vi "Periodic Tasks.vi"(8 "error in":errorcluster) -> ()   [LabVIEW 2019]
doc: "This VI runs in parallel to other tasks. It can contain as many user-defined periodic loops as you need. These can carry out PID or other sorts of timed response."
uses:
  <vilib>/Rock Robotics/WPI/DriverStation/WPI_DriverStationRobotMode2.ctl
  <vilib>/Rock Robotics/WPI/Utilities/WPI_GetSetVariantRefNum.vi
  <vilib>/Rock Robotics/Network Tables/NT Read Boolean.vi
  Robot Global Data.vi
  <vilib>/Rock Robotics/Network Tables/NT Write Boolean.vi
  <vilib>/Rock Robotics/Network Tables/NT Write Number.vi
  <vilib>/Rock Robotics/WPI/RobotDrive/WPI_RobotDriveArcadeDrive_Standard(NoSaturation).vi
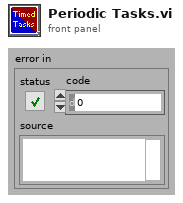
[diagram p1: front panel]
types:
  T1 = typedef "WPI_JoystickDevRef.ctl" = cluster{"Device":T2}
  T2 = typedef "WPI_JoystickDeviceEnum.ctl" = enum16{"USB 0", "USB 1", "USB 2", "USB 3", "USB 4", "USB 5"}
  T3 = typedef "WPI_RobotDriveDevRef.ctl" = cluster{"DevStatus":errorcluster, "Motors[]":T4[], "Square Inputs":bool, "Max Output":dbl}
  T4 = typedef "WPI_MotorControlDeviceRef.ctl" = cluster{"DeviceStatus":errorcluster, "Type":T5, "PWM":cluster{"PWM Channel":T6, "DeadBand":T7}, "CAN":cluster{"Device Number":u8, "SetOutput VI Ref":variant, "GetOutput VI Ref":variant, "Enable VI Ref":variant, "Disable VI Ref":variant, "Data":variant}, "Invert":bool, "DIO PWM":cluster{"PWM \"Enable\" Channel":T6, "DIOChannel":T8, "PWM Rate":dbl}}
  T5 = typedef "WPI_MotorControlType.ctl" = enum16{"PWM", "CAN", "DIO PWM"}
  T6 = typedef "FPGA_DIOPWMChannel.ctl" = enum8{"PWM 0", "PWM 1", "PWM 2", "PWM 3", "PWM 4", "PWM 5", "PWM 6", "PWM 7", "PWM 8", "PWM 9", "PWM MXP 0", "PWM MXP 1", "PWM MXP 2", "PWM MXP 3", "PWM MXP 4", "PWM MXP 5", "PWM MXP 6", "PWM MXP 7", "PWM MXP 8", "PWM MXP 9", "Invalid"}
  T7 = typedef "WPI_PWMDeadband.ctl" = cluster{"Name":string, "maxPositivePwm":i32, "minPositivePwm":i32, "centerPwm":i32, "maxNegativePwm":i32, "minNegativePwm":i32, "angularRange":u16}
  T8 = typedef "FPGA_DIOChannel.ctl" = enum8{"DIO 0", "DIO 1", "DIO 2", "DIO 3", "DIO 4", "DIO 5", "DIO 6", "DIO 7", "DIO 8", "DIO 9", "DIO MXP 0", "DIO MXP 1", "DIO MXP 2", "DIO MXP 3", "DIO MXP 4", "DIO MXP 5", "DIO MXP 6", "DIO MXP 7", "DIO MXP 8", "DIO MXP 9", "DIO MXP 10", "DIO MXP 11", "DIO MXP 12", "DIO MXP 13", "DIO MXP 14", "DIO MXP 15", "SPI Port CS1", "SPI Port CS2", "SPI Port CS3", "SPI Port MISO", "SPI Port MOSI", "Invalid"}
  T9 = cluster{"JoystickDevRef":T1, "RobotDriveDevRef":T3}
  T10 = typedef "WPI_DriverStationRobotMode2.ctl" = enum16{"Autonomous Disabled", "Autonomous Enabled", "Teleop Disabled", "Teleop Enabled", "Disconnected", "Finish", "Test Disabled", "Test Enabled", "Emergency Stopped"}
  T11 = typedef "WPI_ServoDeviceRef.ctl" = cluster{"DeviceStatus":errorcluster, "PWM Channel":T6, "DeadBand":T7}
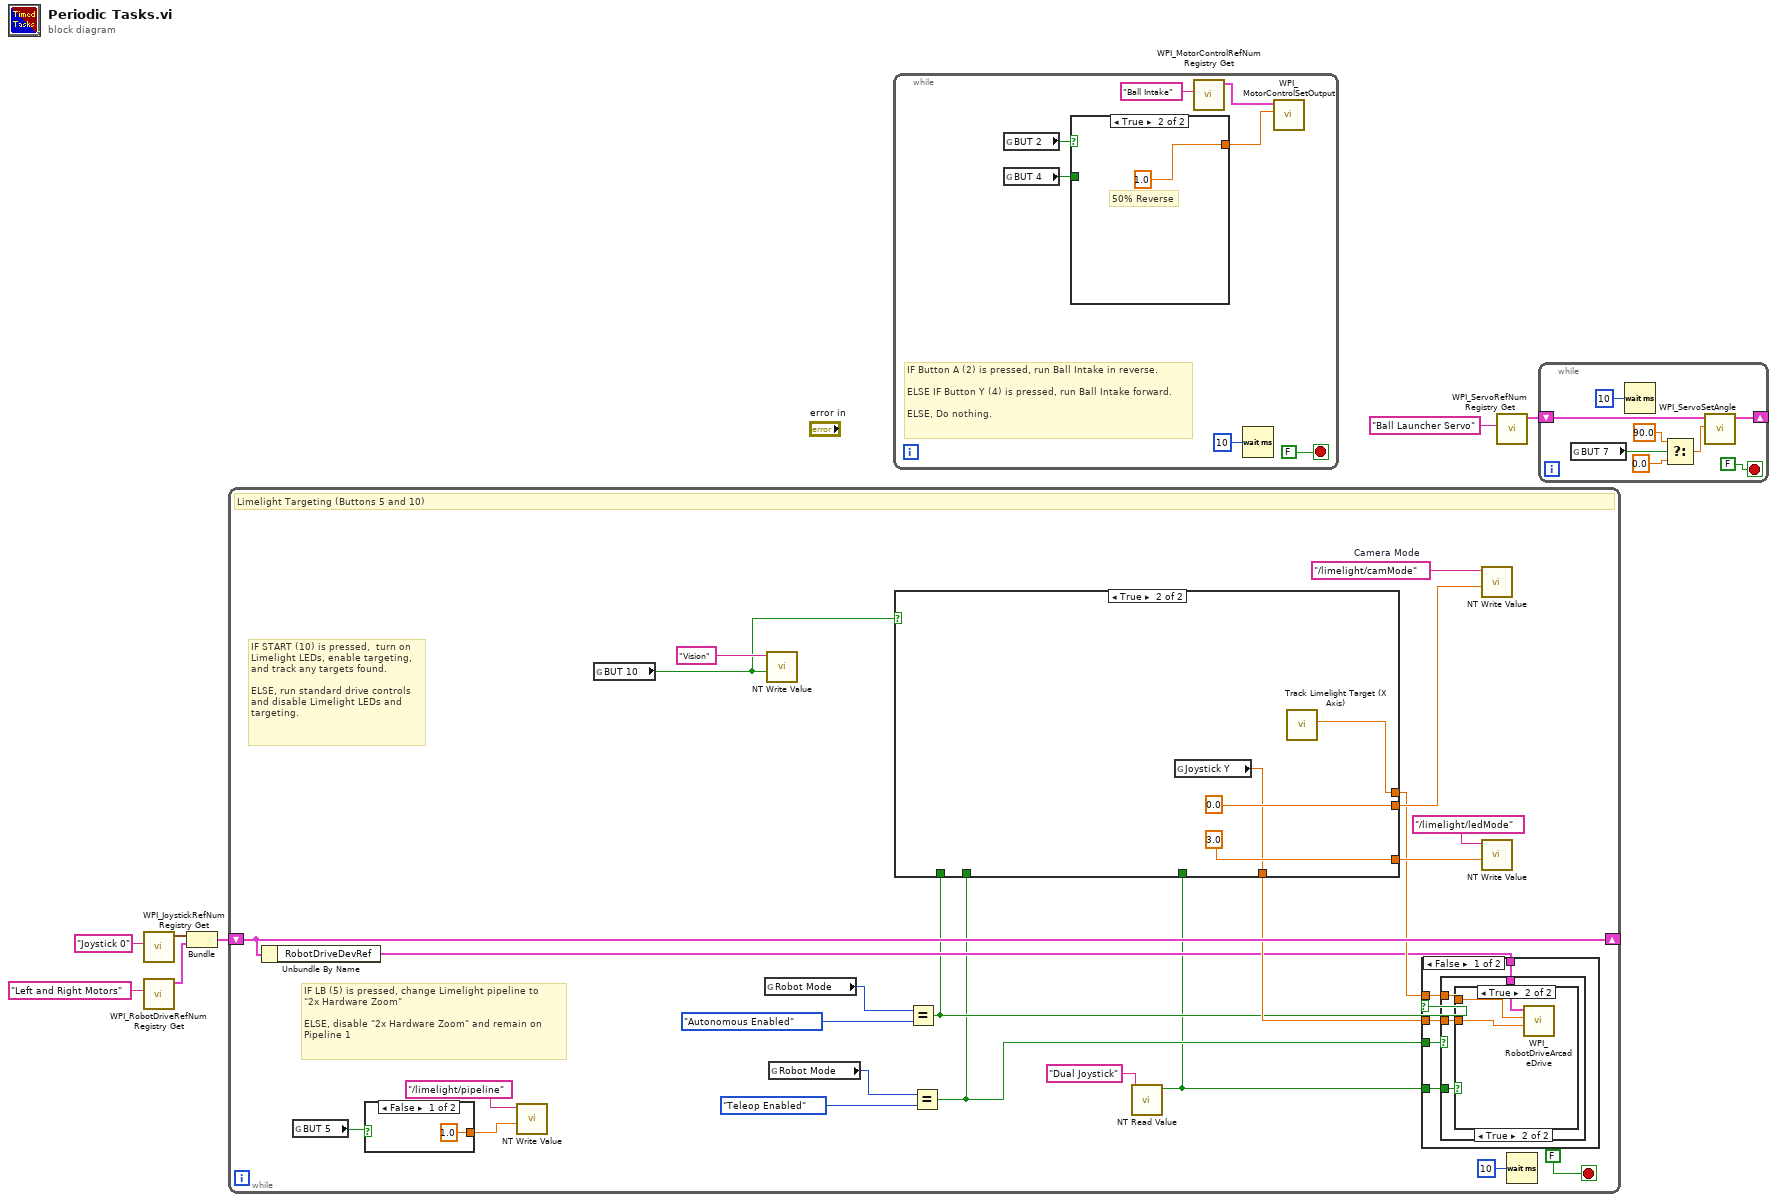
[diagram p0: block diagram]
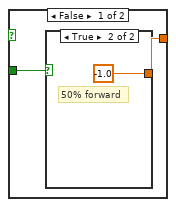
[diagram p2: hidden frame]
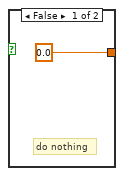
[diagram p3: hidden frame]
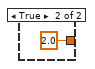
[diagram p4: hidden frame]
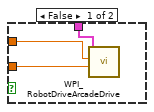
[diagram p5: hidden frame]
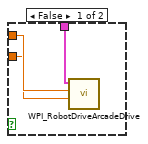
[diagram p6: hidden frame]
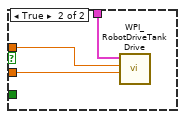
[diagram p7: hidden frame]
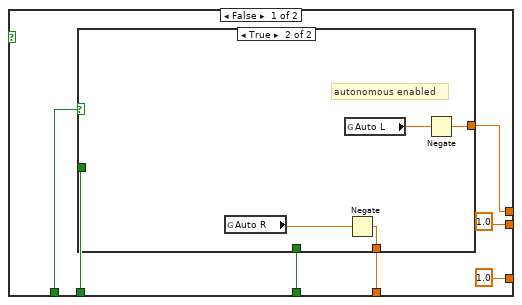
[diagram p8: hidden frame]
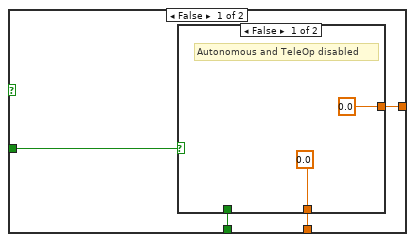
[diagram p9: hidden frame]
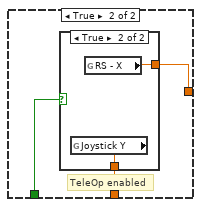
[diagram p10: hidden frame]
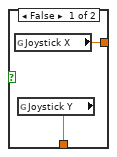
[diagram p11: hidden frame]
diagram:
  n1 = call <vilib>:"WPI_JoystickRefNum Registry Get.vi"("refnum name"="Joystick 0") -> ("JoystickDevRef"=w5:T1)  [unwired: 1 in, 9 out]
  n2 = call <vilib>:"WPI_RobotDriveRefNum Registry Get.vi"("refnum name"="Left and Right Motors") -> ("RobotDriveDevRef"=w4:T3)  [unwired: 1 in, 9 out]
  n3 = Bundle("JoystickDevRef"=w5, "RobotDriveDevRef"=w4) -> (w3:T9)  [unwired: 1 out]
  n4 = while {
    shift-right: [w29] -> _
    shift-left: w3 -> [w29]
    stop <- FALSE stop-if-true
    w27 = "/limelight/camMode"  # Camera Mode
    # "IF LB (5) is pressed, change Limelight pipeline to \n\"2x Hardware Zoom\"\n\nELSE, disable \"2x Hardware Zoom\" and remain on\nPipeline 1"
    # "IF START (10) is pressed,  turn on\nLimelight LEDs, enable targeting,\nand track any targets found.\n\nELSE, run standard drive controls\nand disable Limelight LEDs and \ntargeting."
    # "Limelight Targeting (Buttons 5 and 10)"
    n5 = Unbundle By Name(w29) -> ("RobotDriveDevRef"=w19:T3)
    n6 = global read "Robot Global Data.vi" "BUT 5"() -> (w9:bool)
    n7 = case shown="False" w9 {
      tunnel: [1.0 ("Numeric") 2.0 ("Numeric")] -> w10
      frame False {
      }
      frame True {
      }
    }
    n8 = call-poly <vilib>:"NT Write Value.vi"("Numeric"=w10, "Name"="/limelight/pipeline") -> ()  [unwired: 9 in, 1 out]
    n9 = global read "Robot Global Data.vi" "BUT 10"() -> (w8:bool)
    n10 = global read "Robot Global Data.vi" "Robot Mode"() -> (w18:T10)
    n11 = call-poly <vilib>:"NT Write Value.vi"("Boolean"=w8, "Name"="Vision") -> ()  [unwired: 9 in, 1 out]
    n12 = global read "Robot Global Data.vi" "Robot Mode"() -> (w14:T10)
    n13 = Equal?(x=w18, y=WPI_DriverStationRobotMode2."Autonomous Enabled") -> (x = y?=w16:bool)
    n14 = Equal?(x=w14, y=WPI_DriverStationRobotMode2."Teleop Enabled") -> (x = y?=w13:bool)
    n15 = call-poly <vilib>:"NT Read Value.vi"("Name"="Dual Joystick") -> ("Boolean"=w11:bool)  [unwired: 9 in, 1 out]
    n16 = case shown="True" w8 {
      tunnel: [1.0 ("Numeric") 0.0 ("Numeric")] -> w26
      tunnel: [1.0 ("Numeric") 3.0 ("Numeric")] -> w25
      tunnel: [w57 w79] -> w20
      tunnel: [w58 w78] -> w21
      tunnel: w16 -> [w56 _]
      tunnel: w13 -> [w55 _]
      tunnel: w11 -> [w54 _]
      frame False {
        n17 = case shown="True" w56 {
          tunnel: [w63 w75] -> w58
          tunnel: [w64 w77] -> w57
          tunnel: w55 -> [w62 _]
          tunnel: w54 -> [w61 _]
          frame False {
            n18 = case shown="False" w62 {
              tunnel: [0.0 ("Joystick X") w69] -> w64
              tunnel: [0.0 ("Joystick Y") w68] -> w63
              tunnel: w61 -> [_ w67]
              frame False {
                # "Autonomous and TeleOp disabled"
              }
              frame True {
                # "TeleOp enabled"
                n19 = case shown="True" w67 {
                  tunnel: [w71 w73] -> w69
                  tunnel: [w70 w72] -> w68
                  frame False {
                    n20 = global read "Robot Global Data.vi" "Joystick X"() -> (w71:dbl)
                    n21 = global read "Robot Global Data.vi" "Joystick Y"() -> (w70:dbl)
                  }
                  frame True {
                    n22 = global read "Robot Global Data.vi" "Joystick Y"() -> (w72:dbl)
                    n23 = global read "Robot Global Data.vi" "RS - X"() -> (w73:dbl)
                  }
                }
              }
            }
          }
          frame True {
            # "autonomous enabled"
            n24 = global read "Robot Global Data.vi" "Auto R"() -> (w74:dbl)
            n25 = global read "Robot Global Data.vi" "Auto L"() -> (w76:dbl)
            n26 = Negate(x=w74) -> (-x=w75:dbl)
            n27 = Negate(x=w76) -> (-x=w77:dbl)
          }
        }
      }
      frame True {
        n28 = global read "Robot Global Data.vi" "Joystick Y"() -> (w78:dbl)
        n29 = call "Track Limelight Target (X Axis).vi"() -> ("Joystick X"=w79:dbl)  [unwired: 11 in]
      }
    }
    n30 = case shown="False" w16 {
      tunnel: w21 -> [w37 w51]
      tunnel: w20 -> [w36 w52]
      tunnel: w19 -> [w35 w53]
      tunnel: w13 -> [w34 _]
      tunnel: w11 -> [w33 _]
      frame False {
        n31 = case shown="True" w34 {
          tunnel: w37 -> [w39 w44]
          tunnel: w36 -> [w40 w43]
          tunnel: w35 -> [w38 w42]
          tunnel: w33 -> [_ w41]
          frame False {
            n32 = call-poly <vilib>:"WPI_RobotDriveArcadeDrive.vi"("Y axis value"=w39, "X axis value"=w40, "RobotDriveDevRef"=w38) -> ()  [unwired: 6 in, 3 out]
          }
          frame True {
            n33 = case shown="True" w41 {
              tunnel: w44 -> [w45 w50]
              tunnel: w43 -> [w46 w48]
              tunnel: w42 -> [w47 w49]
              frame False {
                n34 = call-poly <vilib>:"WPI_RobotDriveArcadeDrive.vi"("Y axis value"=w45, "X axis value"=w46, "RobotDriveDevRef"=w47) -> ()  [unwired: 6 in, 3 out]
              }
              frame True {
                n35 = call-poly <vilib>:"WPI_RobotDriveArcadeDrive.vi"("Y axis value"=w50, "X axis value"=w48, "RobotDriveDevRef"=w49) -> ()  [unwired: 6 in, 3 out]
              }
            }
          }
        }
      }
      frame True {
        n36 = call <vilib>:"WPI_RobotDriveTankDrive.vi"("Right axis value"=w51, "Left axis value"=w52, "RobotDriveDevRef"=w53) -> ()  [unwired: 6 in, 3 out]
      }
    }
    n37 = call-poly <vilib>:"NT Write Value.vi"("Numeric"=w26, "Name"=w27) -> ()  [unwired: 9 in, 1 out]
    n38 = call-poly <vilib>:"NT Write Value.vi"("Numeric"=w25, "Name"="/limelight/ledMode" ("LED Mode")) -> ()  [unwired: 9 in, 1 out]
    n39 = Wait (ms)(milliseconds to wait=u32 10) -> ()  [unwired: 1 out]
  }
  n40 = while {
    stop <- FALSE stop-if-true
    # "IF Button A (2) is pressed, run Ball Intake in reverse. \n\nELSE IF Button Y (4) is pressed, run Ball Intake forward.\n\nELSE, Do nothing."
    n41 = global read "Robot Global Data.vi" "BUT 2"() -> (w87:bool)
    n42 = global read "Robot Global Data.vi" "BUT 4"() -> (w86:bool)
    n43 = case shown="True" w87 {
      tunnel: [w90 1.0 ("Output")] -> w88
      tunnel: w86 -> [w89 _]
      frame False {
        n44 = case shown="True" w89 {
          tunnel: [0.0 ("Output") -1.0 ("Output")] -> w90
          frame False {
            # "do nothing"
          }
          frame True {
            # "50% forward"
          }
        }
      }
      frame True {
        # "50% Reverse"
      }
    }
    n45 = call <vilib>:"WPI_MotorControlRefNum Registry Get.vi"("refnum name"="Ball Intake") -> ("MotorControlDevRef"=w84:T4)  [unwired: 9 in, 1 out]
    n46 = Wait (ms)(milliseconds to wait=u32 10) -> ()  [unwired: 1 out]
    n47 = call <vilib>:"WPI_MotorControlSetOutput.vi"("Output"=w88, "MotorControlDevRef"=w84) -> ()  [unwired: 7 in, 3 out]
  }
  n48 = call <vilib>:"WPI_ServoRefNum Registry Get.vi"("refnum name"="Ball Launcher Servo") -> ("ServoDeviceRef"=w1:T11)  [unwired: 9 in, 1 out]
  n49 = while {
    shift-right: [w97] -> _
    shift-left: w1 -> [w96]
    stop <- FALSE stop-if-true
    n50 = global read "Robot Global Data.vi" "BUT 7"() -> (w94:bool)
    n51 = Wait (ms)(milliseconds to wait=u32 10) -> ()  [unwired: 1 out]
    n52 = Select(t=90.0, s=w94, f=0.0) -> (s? t:f=w95:dbl)
    n53 = call <vilib>:"WPI_ServoSetAngle.vi"("Angle"=w95, "ServoDeviceRef"=w96) -> ("ServoDeviceRef"=w97:T11)  [unwired: 8 in, 1 out]
  }
